vi "Tosca-Ramp Down.vi"(0 "Queue in":refnum<queue>, 7 "Stim data in":T1) -> (4 "Queue out":refnum<queue>, 13 "tail":dbl[][](array[numeric]), 15 "error out":errorcluster)   [LabVIEW 2020]
uses:
  Typedefs/Tosca-State AODO.ctl
  epl-vi-lib/Signal Synthesis VIs/4th Generation/Classes/SignalManager/SignalManager.lvclass
  Typedefs/Tosca-AO Runtime.ctl
  Typedefs/Tosca-DO Runtime.ctl
  Typedefs/Tosca-AODO Data.ctl
  epl-vi-lib/Utility VIs/Array Manipulation VIs/Array-Dimensions (2D).vi
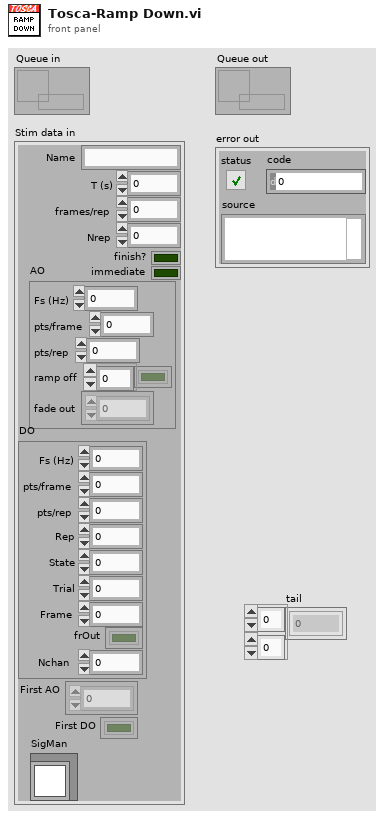
[diagram p1: front panel]
types:
  T1 = typedef "Tosca-State AODO.ctl" = cluster{"Name":string, "T (s)":dbl, "First AO":dbl[][], "frames/rep":i32, "finish?":bool, "Nrep":i32, "AO":T2, "DO":T3, "immediate":bool, "First DO":bool[][], "SigMan":refnum<class "SignalManager.lvclass">}
  T2 = typedef "Tosca-AO Runtime.ctl" = cluster{"Fs (Hz)":dbl, "pts/frame":i32, "pts/rep":i32, "ramp off":bool[], "fade out":dbl[][]}
  T3 = typedef "Tosca-DO Runtime.ctl" = cluster{"Fs (Hz)":dbl, "pts/frame":i32, "pts/rep":i32, "Rep":i32, "State":i32, "Trial":i32, "Frame":i32, "frOut":bool[], "Nchan":i32}
  T4 = typedef "Tosca-AODO Data.ctl" = cluster{"AO":dbl[][], "DO":bool[][], "frame":i32, "stop":bool}
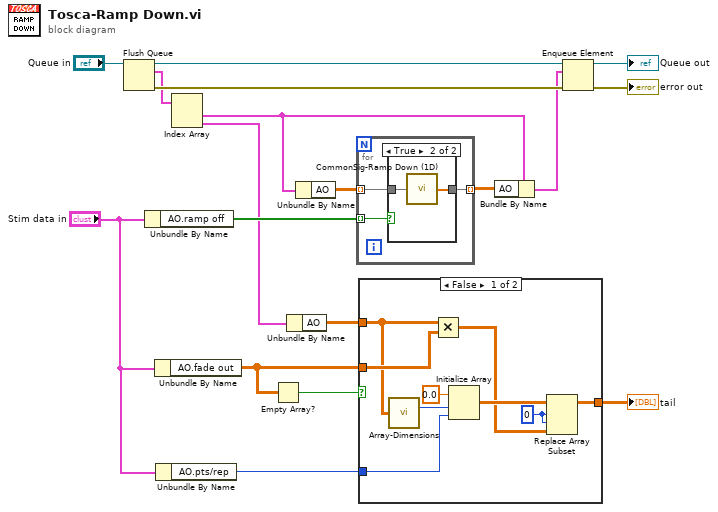
[diagram p0: block diagram]
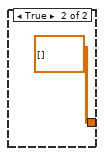
[diagram p2: hidden frame]
diagram:
  n1 = Flush Queue(queue="Queue in") -> (queue out=w15:refnum<queue>, remaining elements=w8:T4[], error out=w14:errorcluster)  [unwired: 1 in]
  n2 = Unbundle By Name("Stim data in") -> ("AO.ramp off"=w17:bool[])
  n3 = Unbundle By Name("Stim data in") -> ("AO.fade out"=w4:dbl[][])
  n4 = Unbundle By Name("Stim data in") -> ("AO.pts/rep"=w2:i32)
  n5 = Index Array(array=w8) -> (element #1=w12:T4, element #2=w7:T4)  [unwired: 2 in]
  n6 = Empty Array?(array=w4) -> (empty?=w6:bool)
  n7 = Unbundle By Name(w7) -> ("AO"=w5:dbl[][])
  n8 = Unbundle By Name(w12) -> ("AO"=w18:dbl[][])
  n9 = for {
    tunnel: w18 -> [w20] mode=indexing
    tunnel: w17 -> [w21] mode=indexing
    tunnel: [w19] -> w16 mode=indexing
    n10 = case shown="True" w21 {
      tunnel: w20 -> [w22 w24]
      tunnel: [w22 w23] -> w19
      frame False {
      }
      frame True {
        n11 = call "CommonSig-Ramp Down (1D).vi"("Array"=w24) -> ("Ramped array"=w23:dbl[])  [unwired: 4 in]
      }
    }
  }
  n12 = case shown="False" w6 {
    tunnel: w5 -> [w27 _]
    tunnel: w4 -> [w33 _]
    tunnel: w2 -> [w32 _]
    tunnel: [w29 dbl[][] []] -> w1
    frame False {
      w30 = 0 ("index (row)")
      n13 = call-poly "Array-Dimensions.vi"("2D Array"=w27) -> ("# rows"=w26:i32)  [unwired: 13 in, 1 out]
      n14 = Multiply(x=w27, y=w33) -> (x*y=w25:dbl[][])
      n15 = Initialize Array(0.0 ("element"), w26, w32) -> (w28:dbl[][])
      n16 = Replace Array Subset(array=w28, new element=w25, index (row)=w30, index (col)=w30) -> (w29:dbl[][])
    }
    frame True {
    }
  }
  "tail" <- w1
  n17 = Bundle By Name(cluster=w12, "AO"=w16) -> (w11:T4)
  n18 = Enqueue Element(queue=w15, element=w11, error in (no error)=w14) -> (queue out=→"Queue out":refnum<queue>, error out=→"error out":errorcluster)  [unwired: 1 in, 1 out]
